vi "Calculate Plot Range.vi"(8 "error in (no error)":errorcluster, 10 "2D Feather Datatype.lvclass in":refnum<class "2D Feather Datatype.lvclass">, 11 "Plot Representation In":T1) -> (0 "error out":errorcluster, 2 "2D Feather Datatype.lvclass out":refnum<class "2D Feather Datatype.lvclass">, 3 "Plot Representation Out":T1)   [LabVIEW 2020, in "2D Feather Datatype.lvclass"]
uses:
  <vilib>/Math Plots/2D Math Plots/2D Feather/2D Feather Datatype/2D Feather Datatype.lvclass
  <vilib>/Math Plots/2D Math Plots/2D Plot/2D Plot/Typedef/Plot Representation.ctl
  <vilib>/Math Plots/2D Math Plots/2D Plot/2D Plot/Typedef/Range Cluster.ctl
  <vilib>/Math Plots/2D Math Plots/2D Plot/2D Plot/2D Plot.lvclass
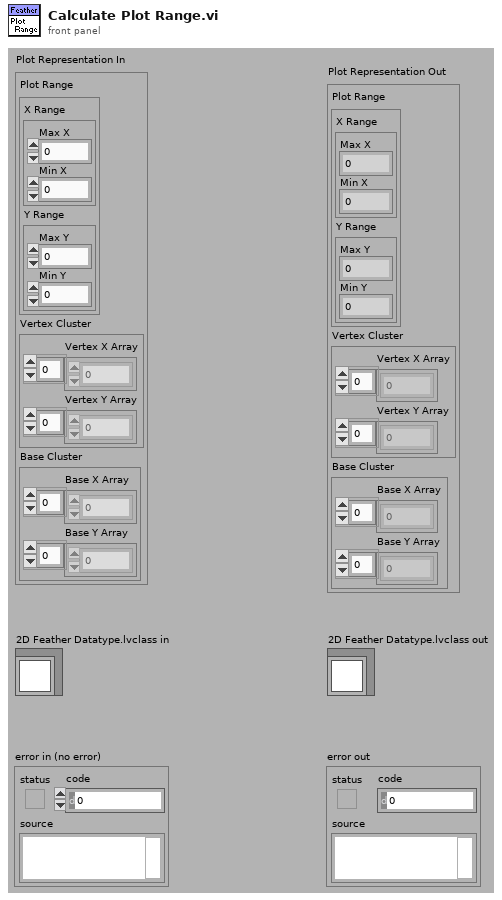
[diagram p1: front panel]
types:
  T1 = typedef "2D Plot.lvclass/Plot Representation.ctl" = cluster{"Plot Range":T2, "Vertex Cluster":cluster{"Vertex X Array":dbl[], "Vertex Y Array":dbl[]}, "Base Cluster":cluster{"Base X Array":dbl[], "Base Y Array":dbl[]}}
  T2 = typedef "2D Plot.lvclass/Range Cluster.ctl" = cluster{"X Range":cluster{"Max X":dbl, "Min X":dbl}, "Y Range":cluster{"Max Y":dbl, "Min Y":dbl}}
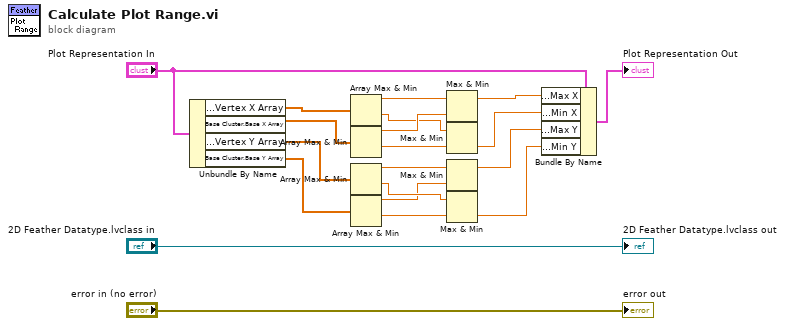
[diagram p0: block diagram]
diagram:
  n1 = Unbundle By Name("Plot Representation In") -> ("Vertex Cluster.Vertex X Array"=w1:dbl[], "Base Cluster.Base X Array"=w2:dbl[], "Vertex Cluster.Vertex Y Array"=w16:dbl[], "Base Cluster.Base Y Array"=w15:dbl[])
  n2 = Array Max & Min(array=w1) -> (max value=w10:dbl, min value=w8:dbl)  [unwired: 2 out]
  n3 = Array Max & Min(array=w2) -> (max value=w9:dbl, min value=w7:dbl)  [unwired: 2 out]
  n4 = Array Max & Min(array=w16) -> (max value=w6:dbl, min value=w5:dbl)  [unwired: 2 out]
  n5 = Array Max & Min(array=w15) -> (max value=w3:dbl, min value=w4:dbl)  [unwired: 2 out]
  n6 = Max & Min(x=w10, y=w9) -> (max(x,y)=w14:dbl)  [unwired: 1 out]
  n7 = Max & Min(x=w8, y=w7) -> (min(x,y)=w13:dbl)  [unwired: 1 out]
  n8 = Max & Min(x=w6, y=w3) -> (max(x,y)=w12:dbl)  [unwired: 1 out]
  n9 = Max & Min(x=w5, y=w4) -> (min(x,y)=w11:dbl)  [unwired: 1 out]
  n10 = Bundle By Name(cluster="Plot Representation In", "Plot Range.X Range.Max X"=w14, "Plot Range.X Range.Min X"=w13, "Plot Range.Y Range.Max Y"=w12, "Plot Range.Y Range.Min Y"=w11) -> (→"Plot Representation Out":T1)
  "2D Feather Datatype.lvclass out" <- "2D Feather Datatype.lvclass in"
  "error out" <- "error in (no error)"
